vi "Create All Message Queues.vi"(7 "QueueName":string, 8 "ErrorIn":errorcluster) -> (0 "ErrorOut":errorcluster, 3 "MessageQueueOut":T1)   [LabVIEW 2016, in "Message Queue.lvlib"]
doc: "Ce VI crée et initialise toutes les files d'attente de messages de l'application. Si votre application nécessite plusieurs files d'attente de messages, cliquez avec le bouton droit sur la constante \"Files d'attente de messages\" et sélectionnez Ouvrir la déf. de type. Ajoutez les nouvelles files d'attente de messages à la définition de type puis initialisez-les dans ce VI."
uses:
  Message Queue.lvlib
  All Message Queues.ctl
  Message Cluster.ctl
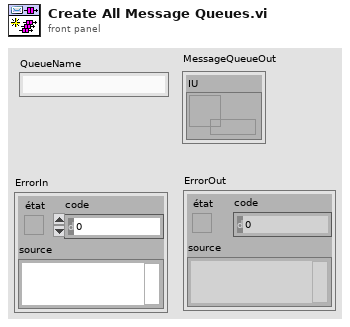
[diagram p1: front panel]
types:
  T1 = typedef "Message Queue.lvlib/All Message Queues.ctl" = cluster{"IU":refnum<queue>}
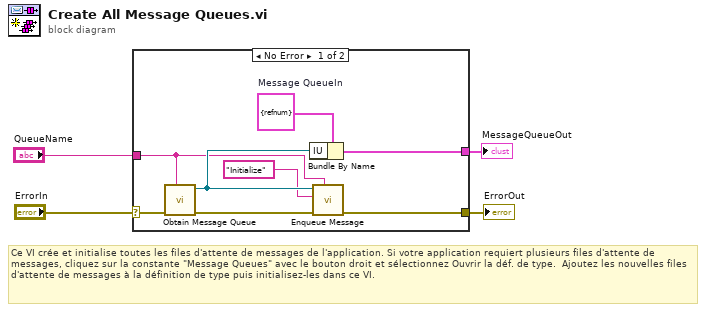
[diagram p0: block diagram]
diagram:
  # "Ce VI crée et initialise toutes les files d'attente de messages de l'application. Si votre application requiert plusieurs files d'attente de messages, cliquez sur la constante \"Message Queues\" avec le bouton droit et sélectionnez Ouvrir la déf. de type.  Ajoutez les nouvelles files d'attente de messages à la définition de type puis initialisez-les dans ce VI."
  n1 = case shown="No Error" "ErrorIn" {
    selector: "ErrorIn" -> [w9 w13]
    tunnel: [w12 w13] -> w4
    tunnel: [w10 _] -> w3
    tunnel: "QueueName" -> [w5 _]
    frame No Error {
      w11 = T1 {"IU"=refnum}  # Message QueueIn
      n2 = call "Obtain Message Queue.vi"("QueueName"=w5, "ErrorIn"=w9) -> ("ErrorOut"=w8:errorcluster, "Message Queue"=w7:refnum<queue>)  [unwired: 8 in]
      n3 = Bundle By Name(cluster=w11, "IU"=w7) -> (w10:T1)
      n4 = call "Enqueue Message.vi"("QueueName"=w5, "error in"=w8, "Message"="Initialize", "Queue"=w7) -> ("error out"=w12:errorcluster)  [unwired: 6 in, 1 out]
    }
    frame Error {
    }
  }
  "MessageQueueOut" <- w3
  "ErrorOut" <- w4
